vi "Debug_visa_close.vi"   [LabVIEW 2015]
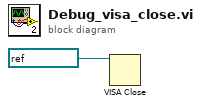
[diagram p0: block diagram]
diagram:
  n1 = VISA Close(VISA resource name=refnum<visa-resource-name> "COM12" ("VISA 리소스 이름")) -> ()  [unwired: 1 in, 1 out]
